vi "All Clear Hover.vi"(8 "error in (no error)":errorcluster, 11 "MCListbox with Checkboxes in":refnum<class "MCListbox with Checkboxes.lvclass">) -> (0 "error out":errorcluster, 3 "MCListbox with Checkboxes out":refnum<class "MCListbox with Checkboxes.lvclass">)   [LabVIEW 2016, in "MCListbox with Checkboxes.lvclass"]
uses:
  MCListbox with Checkboxes.lvclass
  MCListbox with Checkboxes.lvclass/MCListbox with Checkboxes.ctl
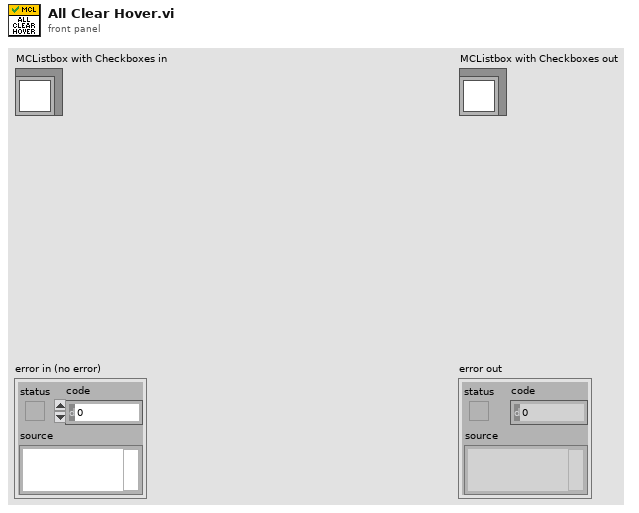
[diagram p1: front panel]
types:
  T1 = cluster{"Symbol (T - Hover)":i32, "Symbol (F - Hover)":i32, "Symbol (T)":i32, "Symbol (F)":i32}
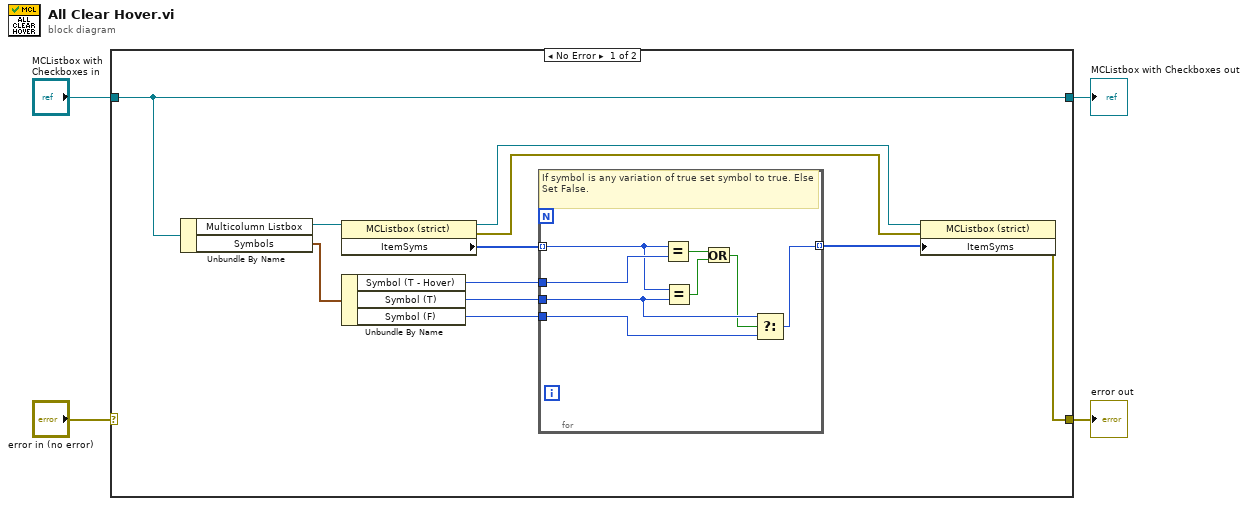
[diagram p0: block diagram]
diagram:
  n1 = case shown="No Error" "error in (no error)" {
    selector: "error in (no error)" -> [_ w25]
    tunnel: [w7 w25] -> w3
    tunnel: [w8 w24] -> w1
    tunnel: "MCListbox with Checkboxes in" -> [w8 w24]
    frame No Error {
      n2 = Unbundle By Name(w8) -> ("Multicolumn Listbox"=w9:refnum<vi>, "Symbols"=w11:T1)
      n3 = property class="MCListbox (strict)"(reference=w9) -> (reference out=w5:refnum<vi>, error out=w6:errorcluster, "ItemSyms"=w10:i32[])  [unwired: 1 in]
      n4 = Unbundle By Name(w11) -> ("Symbol (T - Hover)"=w12:i32, "Symbol (T)"=w13:i32, "Symbol (F)"=w14:i32)
      n5 = for {
        tunnel: w10 -> [w22] mode=indexing
        tunnel: w12 -> [w23]
        tunnel: w13 -> [w21]
        tunnel: w14 -> [w20]
        tunnel: [w19] -> w15 mode=indexing
        # "If symbol is any variation of true set symbol to true. Else Set False."
        n6 = Equal?(x=w22, y=w23) -> (x = y?=w18:bool)
        n7 = Equal?(x=w22, y=w21) -> (x = y?=w17:bool)
        n8 = Or(x=w18, y=w17) -> (x .or. y?=w16:bool)
        n9 = Select(t=w21, s=w16, f=w20) -> (s? t:f=w19:i32)
      }
      n10 = property class="MCListbox (strict)"(reference=w5, error in=w6, "ItemSyms"=w15) -> (error out=w7:errorcluster)  [unwired: 1 out]
    }
    frame Error {
    }
  }
  "error out" <- w3
  "MCListbox with Checkboxes out" <- w1
